vi "Main.vi"(6 "條碼種類":enum16{"EAN", "UPC", "TW_Carrier", "TW_ID"}(ring)) -> ()   [LabVIEW 2026]
uses:
  vision_core_c/bin/barcode_validate.dll
  vision_core_c/bin/barcode_decode.dll
panel:
  in  "Prod_a":enum32{"條碼檢查(bar code)", "數學計算(math)"}(tab)
  in  "圖檔路徑":path
  out "條碼編號":string
  out "編碼正確":bool
  out "Error Code (validate)":i32
  out "Error Code (detect)":i32
  out "讀檔正確":bool
  out "讀檔檢查Error":string
  out "編碼檢查Error":string
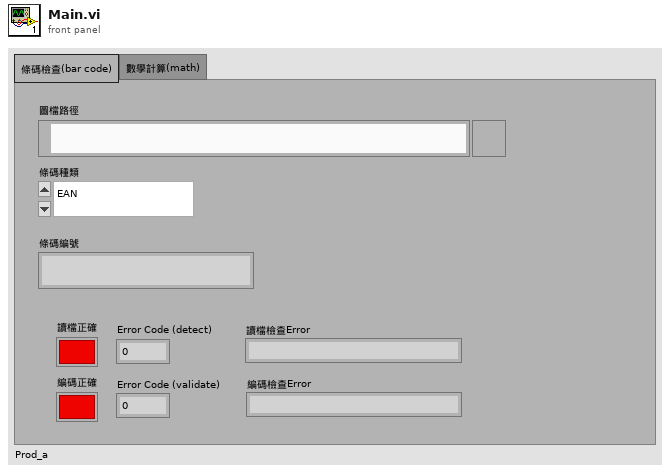
[diagram p1: front panel]
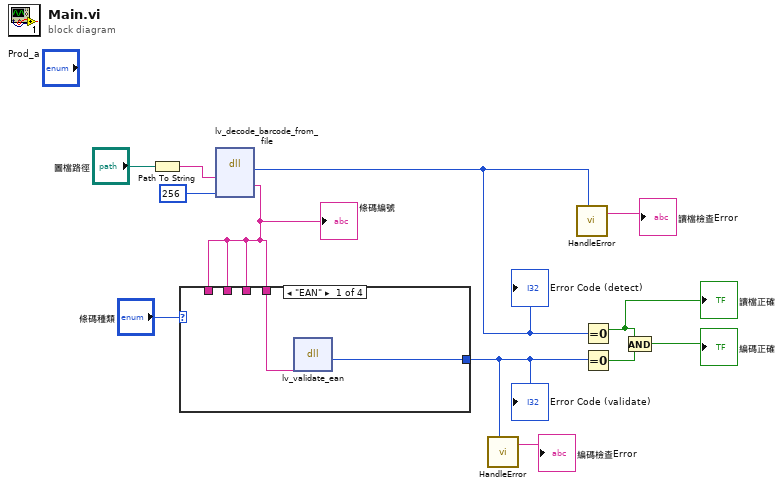
[diagram p0: block diagram]
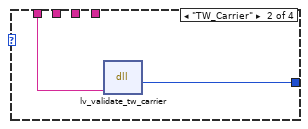
[diagram p2: hidden frame]
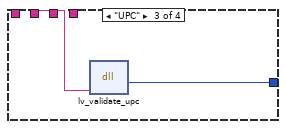
[diagram p3: hidden frame]
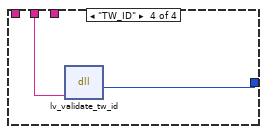
[diagram p4: hidden frame]
diagram:
  n1 = Path To String(path="圖檔路徑") -> (string=w9:string)
  n2 = dll-call lib="D:/git_proj/LabC-Vision/vision_core_c/bin/barcode_decode.dll" fn="lv_decode_barcode_from_file"("image_path"=w9, "out_code_size"=256) -> ("return"=w4:i32, "out_code"=w8:string)  [unwired: 6 in, 2 out]
  "條碼編號" <- w8
  "Error Code (detect)" <- w4
  n3 = case shown="\"EAN\"" "條碼種類" {
    tunnel: w8 -> [_ w16 _ _]
    tunnel: w8 -> [w14 _ _ _]
    tunnel: w8 -> [_ _ w18 _]
    tunnel: w8 -> [_ _ _ w20]
    tunnel: [w13 w15 w17 w19] -> w2
    frame "EAN" {
      n4 = dll-call lib="D:/git_proj/LabC-Vision/vision_core_c/bin/barcode_validate.dll" fn="lv_validate_ean"("code"=w14) -> ("return"=w13:i32)  [unwired: 4 in, 2 out]
    }
    frame "TW_Carrier" {
      n5 = dll-call lib="D:/git_proj/LabC-Vision/vision_core_c/bin/barcode_validate.dll" fn="lv_validate_tw_carrier"("code"=w16) -> ("return"=w15:i32)  [unwired: 4 in, 2 out]
    }
    frame "UPC" {
      n6 = dll-call lib="D:/git_proj/LabC-Vision/vision_core_c/bin/barcode_validate.dll" fn="lv_validate_upc"("code"=w18) -> ("return"=w17:i32)  [unwired: 4 in, 2 out]
    }
    frame "TW_ID" {
      n7 = dll-call lib="D:/git_proj/LabC-Vision/vision_core_c/bin/barcode_validate.dll" fn="lv_validate_tw_id"("code"=w20) -> ("return"=w19:i32)  [unwired: 4 in, 2 out]
    }
  }
  "Error Code (validate)" <- w2
  n8 = call "HandleError.vi"("code"=w2) -> ("out_message"=→"編碼檢查Error":string)  [unwired: 10 in]
  n9 = call "HandleError.vi"("code"=w4) -> ("out_message"=→"讀檔檢查Error":string)  [unwired: 10 in]
  n10 = Equal To 0?(x=w4) -> (x = 0?=w5:bool)
  "讀檔正確" <- w5
  n11 = Equal To 0?(x=w2) -> (x = 0?=w7:bool)
  n12 = And(x=w5, y=w7) -> (x .and. y?=→"編碼正確":bool)
